vi "Command Cube Outtake.vi"(7 "Startup":bool, 11 "Speed":dbl) -> (3 "Output":dbl, 4 "Reinit":bool, 6 "Completed":bool)   [LabVIEW 2017]
uses:
  Command Execution State.ctl
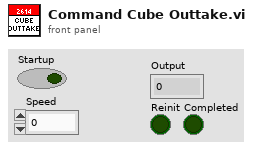
[diagram p1: front panel]
types:
  T1 = typedef "Command Execution State.ctl" = enum16{"Initialize", "Execute", "Finish"}
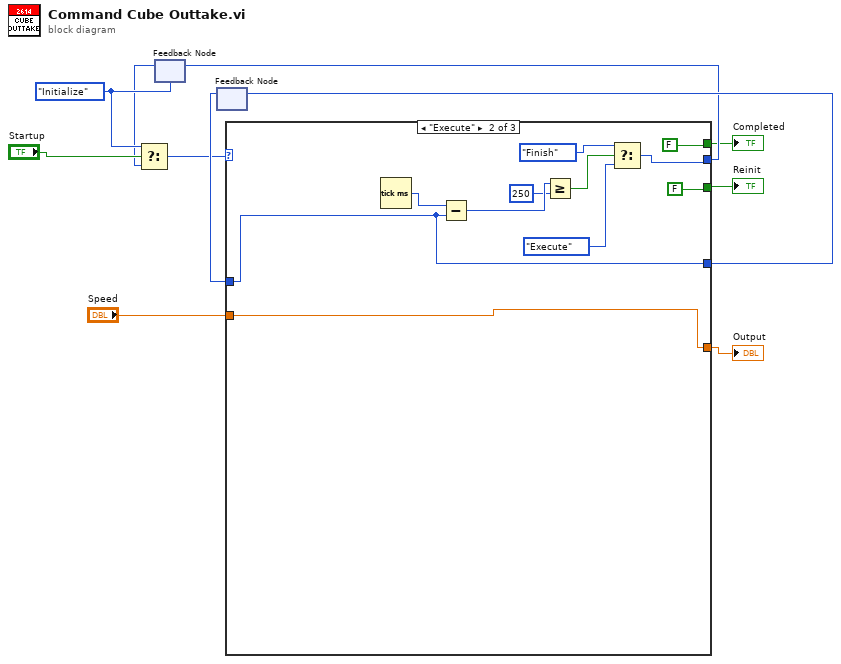
[diagram p0: block diagram]
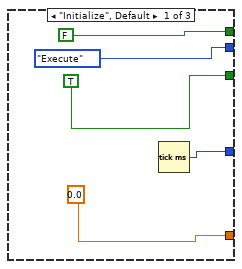
[diagram p2: hidden frame]
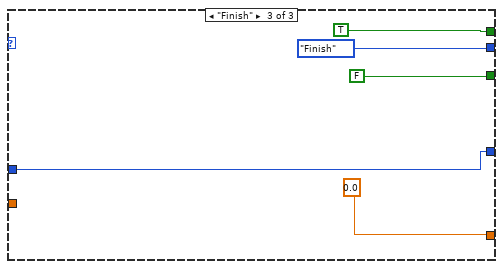
[diagram p3: hidden frame]
diagram:
  w8 = Command_Execution_State."Initialize" ("Play State")
  n1 = feedback #1(w8) -> (w7:T1)
  n2 = Select(t=w8, s="Startup", f=w7) -> (s? t:f=w9:T1)
  n3 = feedback #2() -> (w10:u32)  [unwired: 1 in]
  n4 = case shown="\"Execute\"" w9 {
    tunnel: w10 -> [_ w20 w28]
    tunnel: "Speed" -> [_ w22 _]
    tunnel: [w16 w20 w28] -> w5
    tunnel: [TRUE FALSE FALSE] -> w4
    tunnel: [0.0 w22 0.0] -> w3
    tunnel: [Command_Execution_State."Execute" ("Play State") w25 Command_Execution_State."Finish" ("Play State")] -> w2
    tunnel: [FALSE FALSE TRUE] -> w1
    frame "Initialize", Default {
      n5 = Tick Count (ms)() -> (millisecond timer value=w16:u32)
    }
    frame "Execute" {
      n6 = Tick Count (ms)() -> (millisecond timer value=w21:u32)
      n7 = Subtract(x=w21, y=w20) -> (x-y=w19:u32)
      n8 = Greater Or Equal?(x=w19, y=u32 250) -> (x >= y?=w18:bool)
      n9 = Select(t=Command_Execution_State."Finish" ("Play State"), s=w18, f=Command_Execution_State."Execute" ("Play State")) -> (s? t:f=w25:T1)
    }
    frame "Finish" {
    }
  }
  "Output" <- w3
  "Reinit" <- w4
  "Completed" <- w1
  n10 = feedback-in #1(w2) -> ()
  n11 = feedback-in #2(w5) -> ()
